vi "Write configuration.vi"(8 "error in":errorcluster, 10 "configuration":refnum<class "NISE_CEF_serializable configuration.lvclass">, 11 "Systems in":refnum<class "Systems.lvclass">) -> (0 "error out":errorcluster, 3 "Systems out":refnum<class "Systems.lvclass">)   [LabVIEW 2013, in "PL Framework Configuration Tool.lvlib" / "Systems.lvclass"]
uses:
  Systems.lvclass
  <vilib>/NI/Configuration Framework/serializable configuration/NISE_CEF_serializable configuration.lvclass
  Framework Configuration Classes/system configuration/PL_System Configuration.lvclass
  Systems.lvclass/Systems.ctl
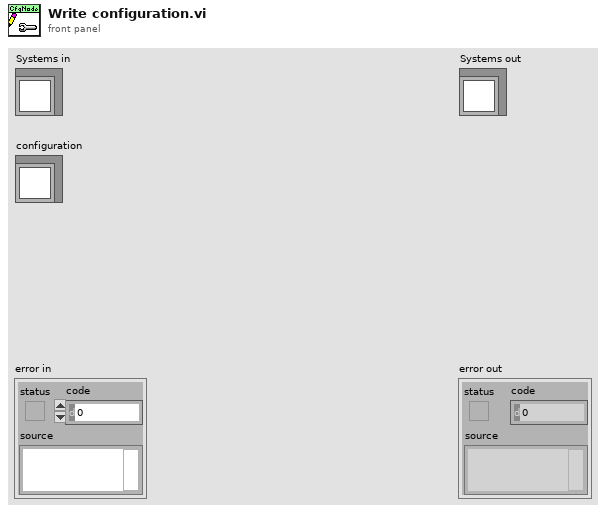
[diagram p1: front panel]
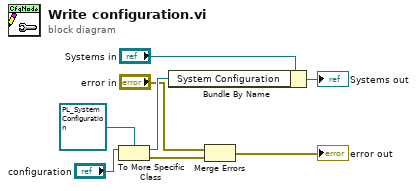
[diagram p0: block diagram]
diagram:
  n1 = To More Specific Class(target class=refnum<class "PL_System Configuration.lvclass"> refnum ("System Configuration"), reference="configuration") -> (specific class reference=w7:refnum<class "PL_System Configuration.lvclass">, error out=w6:errorcluster)  [unwired: 1 in]
  n2 = Bundle By Name(cluster="Systems in", "System Configuration"=w7) -> (→"Systems out":refnum<class "Systems.lvclass">)
  n3 = Merge Errors("error in", w6) -> (→"error out":errorcluster)
